vi "ReadFileContents.vi"(9 "Console":string) -> (0 "File Contents":string, 2 "Success?":bool)   [LabVIEW 2016]
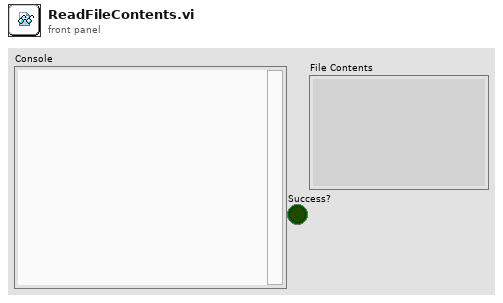
[diagram p1: front panel]
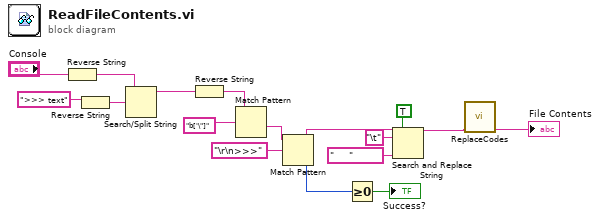
[diagram p0: block diagram]
diagram:
  n1 = Reverse String(1:"Console") -> (0:w12:string)
  n2 = Reverse String(1:">>> text" ("search string/char (-)")) -> (0:w11:string)
  n3 = Search/Split String(string=w12, search string/char (-)=w11) -> (substring before match=w10:string)  [unwired: 1 in, 2 out]
  n4 = Reverse String(1:w10) -> (0:w8:string)
  n5 = Match Pattern(string=w8, regular expression="b['\"]" ("write buffer")) -> (after substring=w15:string)  [unwired: 1 in, 3 out]
  n6 = Match Pattern(string=w15, regular expression="\r\n>>>" ("write buffer")) -> (before substring=w4:string, offset past match=w2:i32)  [unwired: 1 in, 2 out]
  n7 = Greater Or Equal To 0?(x=w2) -> (x >= 0?=→"Success?":bool)
  n8 = Search and Replace String(replace all?=TRUE ("replace all? (F)"), input string=w4, search string="\t", replace string="     " ("replace string (\"\")")) -> (result string=w3:string)  [unwired: 4 in, 3 out]
  n9 = call "ReplaceCodes.vi"("Conv String in"=w3) -> ("String out"=→"File Contents":string)  [unwired: 9 in, 1 out]
